vi "Select Servicio Seleccionado.vi"(8 "error in (no error)":errorcluster, 10 "Servicio Seleccionado":string, 11 "Paquetes in":refnum<class "Paquetes.lvclass">) -> (0 "error out":errorcluster, 3 "Paquetes out":refnum<class "Paquetes.lvclass">)   [LabVIEW 2020, in "Paquetes.lvlib" / "Paquetes.lvclass"]
uses:
  Paquetes.lvclass
  Paquetes.lvclass/Paquetes.ctl
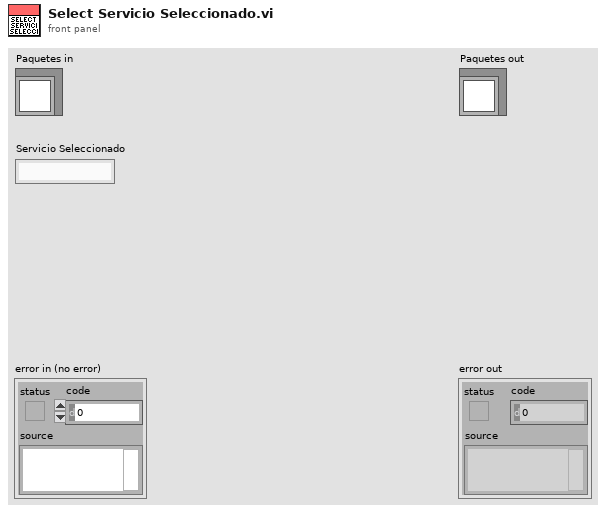
[diagram p1: front panel]
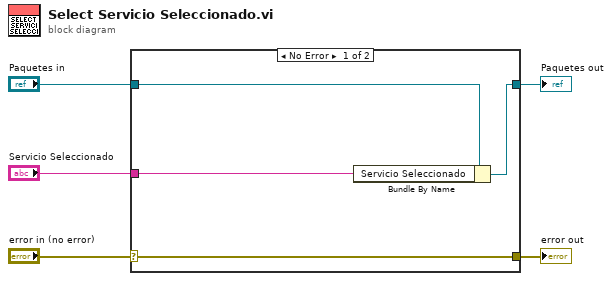
[diagram p0: block diagram]
diagram:
  n1 = case shown="No Error" "error in (no error)" {
    selector: "error in (no error)" -> [w9 w10]
    tunnel: [w9 w10] -> w4
    tunnel: [w7 w11] -> w2
    tunnel: "Paquetes in" -> [w8 w11]
    tunnel: "Servicio Seleccionado" -> [w6 _]
    frame No Error {
      n2 = Bundle By Name(cluster=w8, "Servicio Seleccionado"=w6) -> (w7:refnum<class "Paquetes.lvclass">)
    }
    frame Error {
    }
  }
  "error out" <- w4
  "Paquetes out" <- w2
